vi "UpdatedHighScore.vi"(0 "tdms file":refnum<k34>, 11 "error in (no error)":errorcluster) -> (4 "tdms file out":refnum<k34>, 6 "Names":string[](array[string]), 10 "Scores":string[](array[string]), 15 "error out":errorcluster)   [LabVIEW 2022 SP3]
uses:
  f4964591-22ec-4ef2-89ea-eaaee1989f18.vi
  <vilib>/Comparison/Less/Less Functor/Less Functor.lvclass
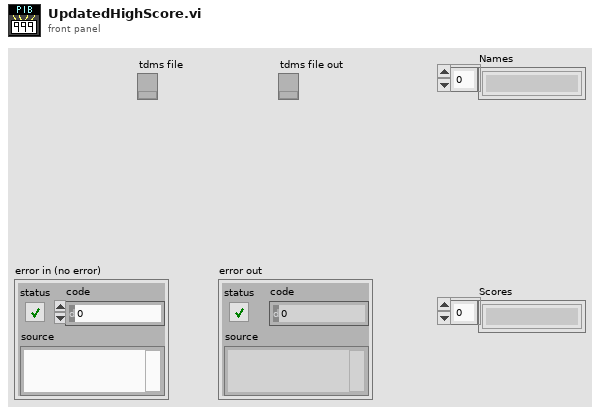
[diagram p1: front panel]
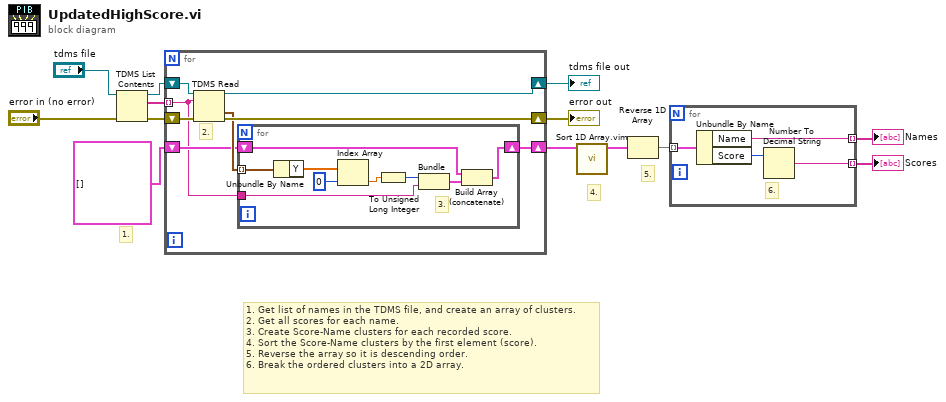
[diagram p0: block diagram]
diagram:
  # "5."
  # "4."
  # "1. Get list of names in the TDMS file, and create an array of clusters.\n2. Get all scores for each name.\n3. Create Score-Name clusters for each recorded score.\n4. Sort the Score-Name clusters by the first element (score).\n5. Reverse the array so it is descending order.\n6. Break the ordered clusters into a 2D array."
  # "1."
  n1 = TDMS List Contents(4:"error in (no error)", 7:"tdms file") -> (0:w11:errorcluster, 2:w13:string[], 3:w12:refnum<k34>)  [unwired: 1 in, 1 out]
  n2 = for {
    shift-right: [w19] -> w2
    shift-left: w12 -> [w21]
    shift-right: [w18] -> w3
    shift-left: w11 -> [w20]
    tunnel: w13 -> [w15] mode=indexing
    shift-right: [w14] -> w9
    shift-left: cluster{"Score":u32, "Name":string}[] [] -> [w16]
    # "2."
    n3 = TDMS Read(0:w21, 5:w15, 11:w20) -> (4:w19:refnum<k34>, 10:w17:waveform(dbl)[], 15:w18:errorcluster)  [unwired: 5 in, 3 out]
    n4 = for {
      tunnel: w17 -> [w30] mode=indexing
      shift-right: [w22] -> w14
      shift-left: w16 -> [w26]
      tunnel: w15 -> [w24]
      # "3."
      n5 = Unbundle By Name(w30) -> ("Y"=w29:dbl[])
      n6 = Index Array(array=w29, index=0) -> (element=w27:dbl)
      n7 = To Unsigned Long Integer(number=w27) -> (unsigned 32bit integer=w25:u32)
      n8 = Bundle(w25, w24) -> (w23:cluster{u32, string})  [unwired: 1 in]
      n9 = Build Array (concatenate)(w26, w23) -> (w22:cluster{"Score":u32, "Name":string}[])
    }
  }
  "error out" <- w3
  "tdms file out" <- w2
  n10 = call "Sort 1D Array.vim"("unsorted array"=w9) -> ("sorted array"=w8:cluster{"Score":u32, "Name":string}[])  [unwired: 10 in]
  n11 = Reverse 1D Array(array=w8) -> (reversed array=w7:cluster{"Score":u32, "Name":string}[])
  n12 = for {
    tunnel: w7 -> [w34] mode=indexing
    tunnel: [w32] -> w6 mode=indexing
    tunnel: [w31] -> w1 mode=indexing
    # "6."
    n13 = Unbundle By Name(w34) -> ("Name"=w32:string, "Score"=w33:u32)
    n14 = Number To Decimal String(number=w33) -> (decimal integer string=w31:string)  [unwired: 1 in]
  }
  "Scores" <- w1
  "Names" <- w6
